vi "HTS_CAVRO_COMMAND_STRING.vi"(2 "Prior Command":string, 5 "PUMP COMMAND":T1, 6 "Parameter <n>":i32) -> (3 "New Command":string)   [LabVIEW 2009]
uses:
  HTS_CAVRO_COMMAND_TYPE.ctl
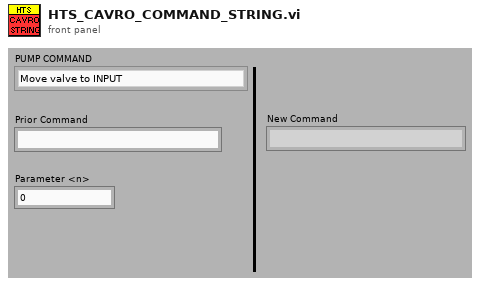
[diagram p1: front panel]
types:
  T1 = typedef "HTS_CAVRO_COMMAND_TYPE.ctl" = enum16{"Move valve to INPUT", "Move valve to INPUT <n>", "Move valve to OUTPUT", "Move valve to OUTPUT <n>", "Move valve to BYPASS", "Move valve to EXTRA", "Syringe to ABSOLUTE  <n>", "Syringe RELATIVE Pickup <n>", "Syringe RELATIVE Dispense <n>", "Set START SPEED <n>", "Set TOP SPEED <n>", "Set CUTOFF in pulses/sec <n>", "Set CUTOFF in increments <n>", "Set SLOPE <n>", "Loop START", "Loop END <n>", "Set AUX OUTPUT <n>", "Delay Command Execution <n>", "EXECUTE COMMAND"}
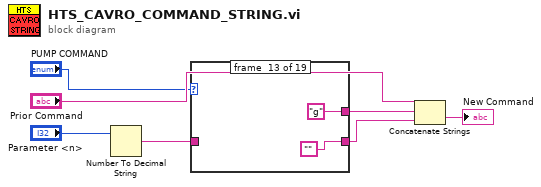
[diagram p0: block diagram]
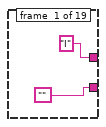
[diagram p2: hidden frame]
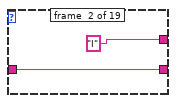
[diagram p3: hidden frame]
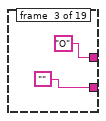
[diagram p4: hidden frame]
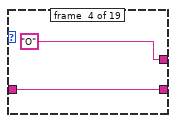
[diagram p5: hidden frame]
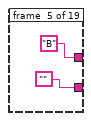
[diagram p6: hidden frame]
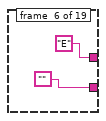
[diagram p7: hidden frame]
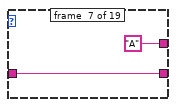
[diagram p8: hidden frame]
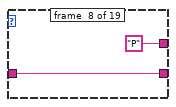
[diagram p9: hidden frame]
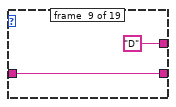
[diagram p10: hidden frame]
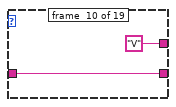
[diagram p11: hidden frame]
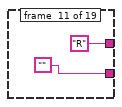
[diagram p12: hidden frame]
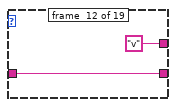
[diagram p13: hidden frame]
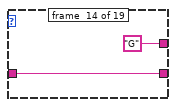
[diagram p14: hidden frame]
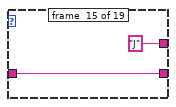
[diagram p15: hidden frame]
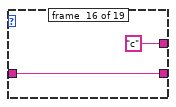
[diagram p16: hidden frame]
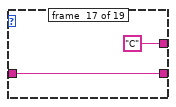
[diagram p17: hidden frame]
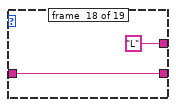
[diagram p18: hidden frame]
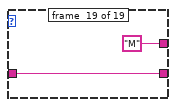
[diagram p19: hidden frame]
diagram:
  n1 = Number To Decimal String(number="Parameter <n>") -> (decimal integer string=w5:string)  [unwired: 1 out]
  n2 = case shown="\"Delay Command Execution <n>\"" "PUMP COMMAND" {
    tunnel: ["I" "I" ("string") "O" "O" ("string") "B" "E" "A" "P" ("string") "D" ("string") "V" ("string") "R" ("string") "v" ("string") "g" ("string") "G" ("string") "J" ("string") "c" ("string") "C" ("string") "L" ("string") "M" ("string")] -> w3
    tunnel: w5 -> [_ w10 _ w14 _ _ w20 w22 w24 w26 _ w31 _ w35 w37 w39 w41 w43 w45]
    tunnel: ["" w10 "" w14 "" "" w20 w22 w24 w26 "" w31 "" w35 w37 w39 w41 w43 w45] -> w7
    frame #0 {
    }
    frame #1 {
    }
    frame #2 {
    }
    frame #3 {
    }
    frame #4 {
    }
    frame #5 {
    }
    frame #6 {
    }
    frame #7 {
    }
    frame #8 {
    }
    frame #9 {
    }
    frame #10 {
    }
    frame #11 {
    }
    frame #12 {
    }
    frame #13 {
    }
    frame #14 {
    }
    frame #15 {
    }
    frame #16 {
    }
    frame #17 {
    }
    frame #18 {
    }
  }
  n3 = Concatenate Strings("Prior Command", w3, w7) -> (→"New Command":string)
